vi "Initialize Kalman Filter.vi"(0 "EKF_Settings":T1={"Gravity constant"=-9.808205458883663, "Filter Version"=enum."IMU, Pressure, Compass", "Initial Biases"={"Gyro_Bias_nit_x"=0.00198, "Gyro_Bias_init_y"=0.0053, "Gyro_Bias_init_z"=0.0009, "Acc_Bias_init_x"=0.0, "Acc_Bias_init_y"=0.0, "Acc_Bias_init_z"=0.0}, "Use Compass on initialisation"=TRUE, "Initial Biases Covariances"={"Initial_covariance_Gyro_Bias"=0.0014, "Initial_covariance_Acc_Bias"=0.2}, "Magnetic-Field-Vector [utesla]"={"Magf_N_x"=21.565, "Magf_N_y"=0.6833, "Magf_N_z"=42.6149}, "IMU_Sigmas"={"Sigma_w"=0.00033937, "Sigma_wb"=3.8785e-05, "Sigma_a"=0.02, "Sigma_ab"=0.03, "Sigma_m"=1000.0}, "Measurement Sigmas"={"Sigma_v"=500.0, "Sigma_depth"=0.2}}, 1 "error in":errorcluster) -> (2 "x_init":dbl[](array[numeric]), 3 "P_init":dbl[][](array[numeric]), 4 "error Out":errorcluster)   [LabVIEW 2013]
uses:
  Controls/EKF_Settings.ctl
  myRIO/Sensors/IMU/IMU_Data_Type_Def.ctl
  <vilib>/Analysis/Matrix/Numeric/Conversions/Array To Matrix - RA.vi
  <vilib>/imath/engines/lvmath2/RunTimeEngine/ErrorHandling/NIMS_Finalize Error.vi
  <vilib>/imath/engines/lvmath2/RunTimeEngine/Managers/WorkSpace/UID Generator.vi
  <vilib>/Analysis/Matrix/Numeric/Conversions/Matrix To Array - RM.vi
  <vilib>/imath/engines/lvmath2/RunTimeEngine/Managers/SymbolTable/Clear UID.vi
  <vilib>/imath/engines/lvmath2/RunTimeEngine/NodeEndStatement/NIMS_NodeEndStatement_Output.vi
  <instcachedir>/0/NIMS_NodeEndStatement_Output_53EC0D466D134D7ABD903AC30B43404B.lvgen/NIMS_NodeEndStatement_Output_53EC0D466D134D7ABD903AC30B43404B_005.vi
  <instcachedir>/0/NIMS_NodeEndStatement_Output_53EC0D466D134D7ABD903AC30B43404B.lvgen/NIMS_NodeEndStatement_Output_53EC0D466D134D7ABD903AC30B43404B_002.vi
  LabVIEW Data/MathScriptVIs/MCStatic_31886544032_abdee02eadfb47e8f2c9b8974125492a.vi
  <instcachedir>/0/MCStatic_31886544032_abdee02eadfb47e8f2c9b8974125492a_9BDEF84E621C4F959353EF47A14DF286.lvgen/MCStatic_31886544032_abdee02eadfb47e8f2c9b8974125492a_9BDEF84E621C4F959353EF47A14DF286_000.vi
  <vilib>/imath/engines/lvmath2/RunTimeEngine/RunTimeType/NIMS_RunTimeType_From StrictType (excl LVString).vi
  <instcachedir>/0/NIMS_RunTimeType_From StrictType (excl LVString)_4DEE718D6EB74582AA20236969C084FC.lvgen/NIMS_RunTimeType_From StrictType (excl LVString)_4DEE718D6EB74582AA20236969C084FC_000.vi
  <vilib>/imath/engines/lvmath2/RunTimeEngine/LocalVariableDefStatement/MC_LocalVariableDefStatement_Display.vi
  Kalman_Estimator_Matlab_Sepios/matlab_tools/kalman_filter/extended_kalman_filter_process_p_c_init.m
  Kalman_Estimator_Matlab_Sepios/matlab_tools/quaternion/q_min.m
  Kalman_Estimator_Matlab_Sepios/matlab_tools/quaternion/q_mul.m
  Kalman_Estimator_Matlab_Sepios/matlab_tools/quaternion/q_q2R.m
  Kalman_Estimator_Matlab_Sepios/matlab_tools/quaternion/q_q2rpy.m
  Kalman_Estimator_Matlab_Sepios/matlab_tools/quaternion/q_R2q.m
  Kalman_Estimator_Matlab_Sepios/matlab_tools/quaternion/q_rpy2q.m
  Kalman_Estimator_Matlab_Sepios/matlab_tools/quaternion/skewOp.m
  <vilib>/Analysis/Matrix/NI_Matrix.lvlib
  <vilib>/imath/engines/lvmath2/RunTimeEngine/Managers/SymbolTable/NIMS_WorkSpace.lvlib
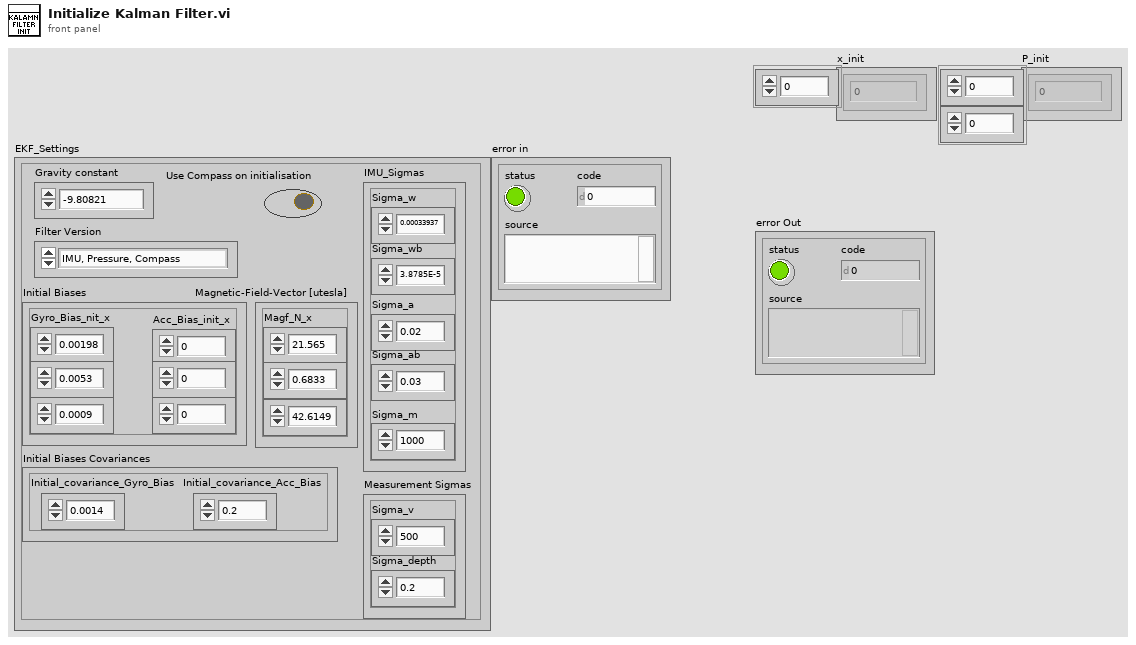
[diagram p1: front panel]
types:
  T1 = typedef "EKF_Settings.ctl" = cluster{"Gravity constant":dbl, "Filter Version":enum16{"IMU Only", "IMU & Pressure", "IMU, Pressure, Compass"}, "Initial Biases":cluster{"Gyro_Bias_nit_x":dbl, "Gyro_Bias_init_y":dbl, "Gyro_Bias_init_z":dbl, "Acc_Bias_init_x":dbl, "Acc_Bias_init_y":dbl, "Acc_Bias_init_z":dbl}, "Use Compass on initialisation":bool, "Initial Biases Covariances":cluster{"Initial_covariance_Gyro_Bias":dbl, "Initial_covariance_Acc_Bias":dbl}, "Magnetic-Field-Vector [utesla]":cluster{"Magf_N_x":dbl, "Magf_N_y":dbl, "Magf_N_z":dbl}, "IMU_Sigmas":cluster{"Sigma_w":dbl, "Sigma_wb":dbl, "Sigma_a":dbl, "Sigma_ab":dbl, "Sigma_m":dbl}, "Measurement Sigmas":cluster{"Sigma_v":dbl, "Sigma_depth":dbl}}
  T2 = typedef "IMU_Data_Type_Def.ctl" = cluster{timestamp, "X_Gyro_Out":dbl, "Y_Gyro_Out":dbl, "Z_Gyro_Out":dbl, "X_Accl_Out":dbl, "Y_Accl_Out":dbl, "Z_Accl_Out":dbl, "X_Magn_Out":dbl, "Y_Magn_Out":dbl, "Z_Magn_Out":dbl, "Temp_Out":dbl, "Barom_Out":dbl}
  T3 = cluster{"Gyro_Bias_nit_x":dbl, "Gyro_Bias_init_y":dbl, "Gyro_Bias_init_z":dbl, "Acc_Bias_init_x":dbl, "Acc_Bias_init_y":dbl, "Acc_Bias_init_z":dbl}
  T4 = cluster{"Initial_covariance_Gyro_Bias":dbl, "Initial_covariance_Acc_Bias":dbl}
  T5 = typedef "NI_Matrix.lvlib/RealMatrix.ctl" = dbl[][]
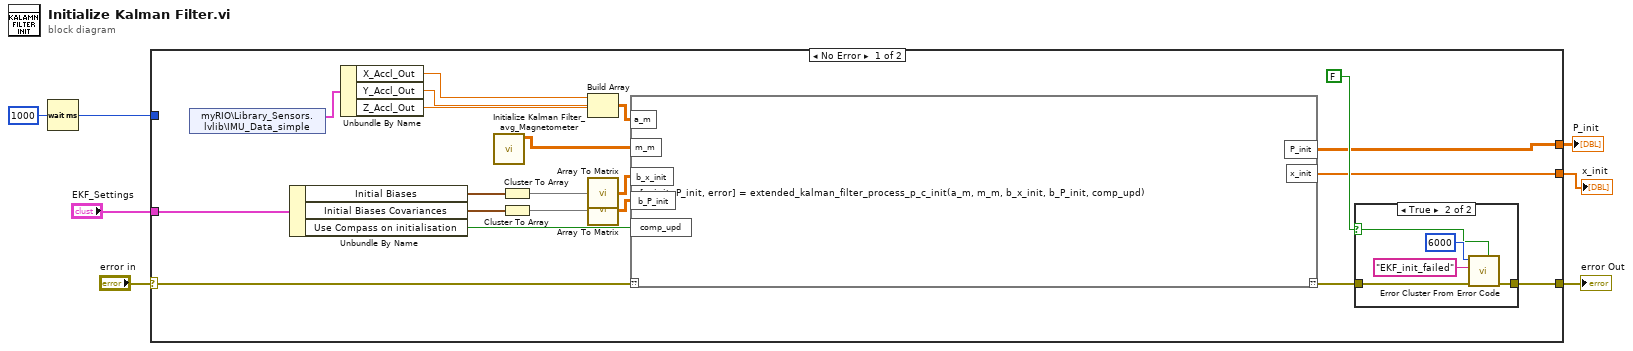
[diagram p0: block diagram]
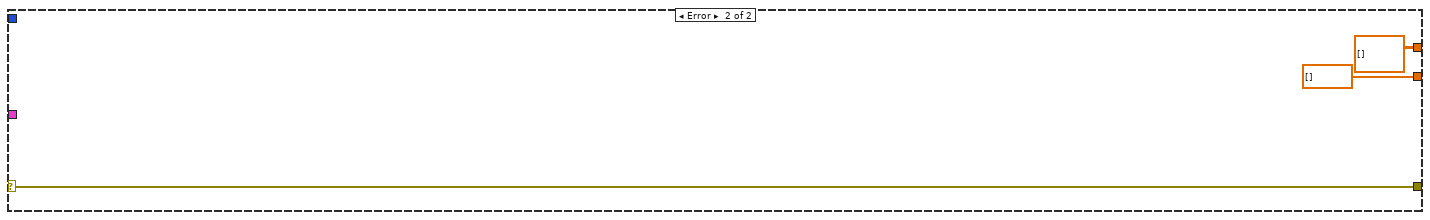
[diagram p3: hidden frame]
diagram:
  n1 = Wait (ms)(milliseconds to wait=u32 1000) -> (millisecond timer value=w1:u32)
  n2 = case shown="No Error" "error in" {
    selector: "error in" -> [w18 w108]
    tunnel: "EKF_Settings" -> [w22 _]
    tunnel: [w16 w108] -> w5
    tunnel: [w10 dbl[][] [] ("P_init")] -> w3
    tunnel: [w9 dbl[] [] ("x_init")] -> w4
    tunnel: w1 -> [_ _]
    frame No Error {
      n3 = shared-variable "myRIO\\Library_Sensors.lvlib\\IMU_Data_simple"() -> (w27:T2)  [unwired: 1 in, 1 out]
      n4 = Unbundle By Name(w22) -> ("Initial Biases"=w21:T3, "Initial Biases Covariances"=w20:T4, "Use Compass on initialisation"=w19:bool)
      n5 = Unbundle By Name(w27) -> ("X_Accl_Out"=w24:dbl, "Y_Accl_Out"=w25:dbl, "Z_Accl_Out"=w26:dbl)
      n6 = call "Initialize Kalman Filter_avg_Magnetometer.vi"() -> ("Averaged Magnetometer-readings"=w8:T5)  [unwired: 11 in]
      n7 = Cluster To Array(cluster=w21) -> (array=w14:dbl[])
      n8 = Cluster To Array(cluster=w20) -> (array=w13:dbl[])
      n9 = Build Array(w24, w25, w26) -> (w23:T5)
      n10 = call-poly <vilib>:"Array To Matrix.vi"("Real 1D Array"=w14) -> ("Real Matrix (Column Vector)"=w12:T5)
      n11 = call-poly <vilib>:"Array To Matrix.vi"("Real 1D Array"=w13) -> ("Real Matrix (Column Vector)"=w11:T5)
      n12 = mathscript code="[x_init, P_init, error] = extended_kalman_filter_process_p_c_init(a_m, m_m, b_x_init, b_P_init, comp_upd)"("??"=w18, "a_m"=w23, "m_m"=w8, "b_x_init"=w12, "b_P_init"=w11, "comp_upd"=w19) -> ("??"=w17:errorcluster, "P_init"=w10:dbl[][], "x_init"=w9:dbl[])
      n13 = case shown="True" FALSE {
        selector: FALSE -> [_ w29]
        tunnel: w17 -> [w28 w31]
        tunnel: [w28 w30] -> w16
        frame False {
        }
        frame True {
          n14 = call <vilib>:"Error Cluster From Error Code.vi"("is warning? (False)"=w29, "error in (no error)"=w31, "error message (\"\")"="EKF_init_failed" ("error message (\"\")"), "error code (0)"=6000) -> ("error out"=w30:errorcluster)  [unwired: 5 in]
        }
      }
    }
    frame Error {
    }
  }
  "error Out" <- w5
  "x_init" <- w4
  "P_init" <- w3
